vi "Bind I16 parameter.vi"(4 "error in (no error)":errorcluster, 6 "Parameter":i16, 7 "Statement Refnum":T1) -> (0 "error out":errorcluster, 3 "Statement Refnum":T1)   [LabVIEW 2011]
doc: "Charge le paramètre de type entier (I16) dans la pile"
uses:
  SQL Controls/Statement Refnum.ctl
  Odbc32.dll
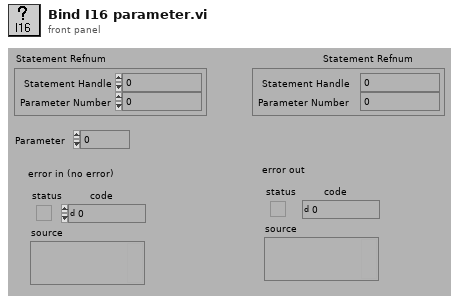
[diagram p1: front panel]
types:
  T1 = typedef "Statement Refnum.ctl" = cluster{"Statement Handle":i32, "Parameter Number":u16}
  T2 = enum16{"NOPE", "SQL_HANDLE_ENV", "SQL_HANDLE_DBC", "SQL_HANDLE_STMT", "SQL_HANDLE_DESC"}
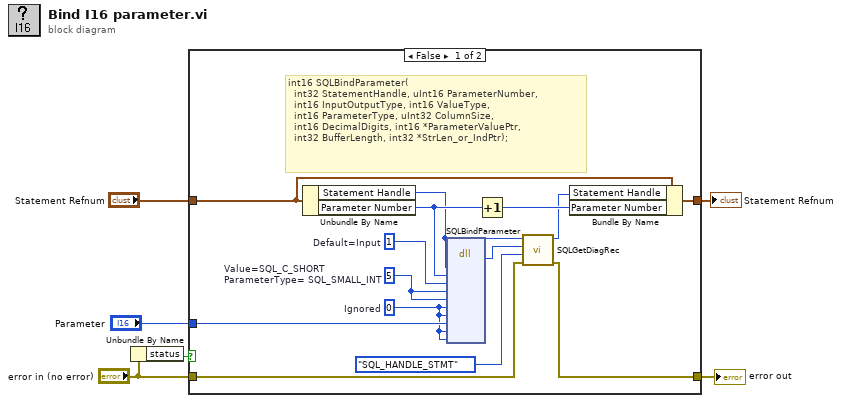
[diagram p0: block diagram]
diagram:
  n1 = Unbundle By Name("error in (no error)") -> ("status"=w1:bool)
  n2 = case shown="False" w1 {
    tunnel: "Parameter" -> [w20 _]
    tunnel: "Statement Refnum" -> [w19 w22]
    tunnel: [w18 w22] -> w4
    tunnel: [w10 w21] -> w3
    tunnel: "error in (no error)" -> [w8 w21]
    frame False {
      w13 = i16 5  # Value=SQL_C_SHORT ParameterType= SQL_SMALL_INT
      w14 = 0  # Ignored
      w16 = i16 1  # Default=Input
      # "int16 SQLBindParameter(\n  int32 StatementHandle, uInt16 ParameterNumber, \n  int16 InputOutputType, int16 ValueType, \n  int16 ParameterType, uInt32 ColumnSize, \n  int16 DecimalDigits, int16 *ParameterValuePtr,\n  int32 BufferLength, int32 *StrLen_or_IndPtr);"
      n3 = Unbundle By Name(w19) -> ("Statement Handle"=w12:i32, "Parameter Number"=w17:u16)
      n4 = dll-call lib="Odbc32.dll" fn="SQLBindParameter"("StatementHandle"=w12, "ParameterNumber"=w17, "InputOutputType"=w16, "ValueType"=w13, "ParameterType"=w13, "ColumnSize"=w14, "DecimalDigits"=w14, "ParameterValuePtr"=w20, "BufferLength"=w14, "StrLen_or_IndPtr"=w14) -> (w9:i16)  [unwired: 11 in, 4 out]
      n5 = Increment(x=w17) -> (x+1=w15:u16)
      n6 = call "SQLGetDiagRec.vi"("error in (no error)"=w8, "HandleType"=T2."SQL_HANDLE_STMT", "Status (SQL_SUCCESS=0)"=w9, "Input Handle"=w12) -> ("error out"=w10:errorcluster, "Output Handle"=w11:i32)  [unwired: 2 out]
      n7 = Bundle By Name(cluster=w19, "Statement Handle"=w11, "Parameter Number"=w15) -> (w18:T1)
    }
    frame True {
    }
  }
  "Statement Refnum" <- w4
  "error out" <- w3
